vi "StopControl.vi"(6 "Loop Iteration":i32, 8 "Reset":bool, 9 "Rate (unit/s)":dbl=0.5, 11 "Motor Value":dbl step=0.1) -> (0 "Done Stopping":bool, 3 "New Motor Value":dbl)   [LabVIEW 2012]
doc: "Stops a given motor value based on time since last call and given rate. Rate of change is always linear with respect to time. Designed to be run multiple times in while loop. Use shift register to maintain Motor Value in external while loop."
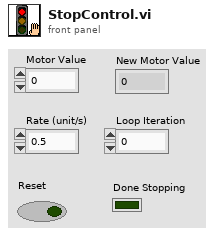
[diagram p1: front panel]
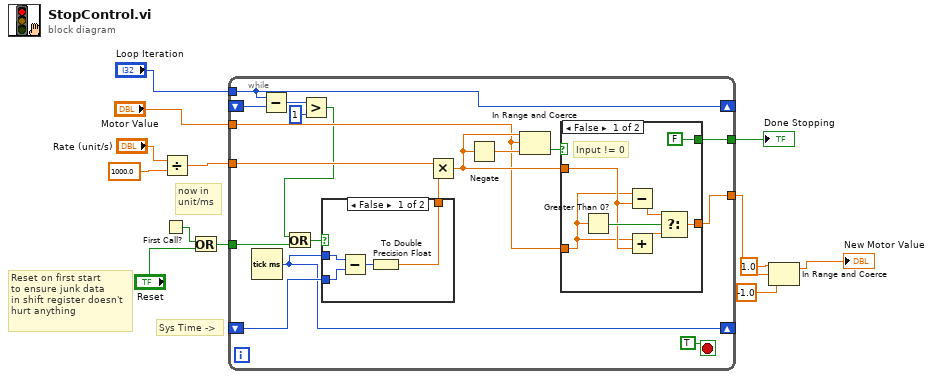
[diagram p0: block diagram]
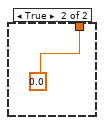
[diagram p2: hidden frame]
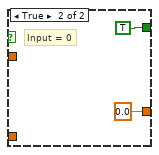
[diagram p3: hidden frame]
diagram:
  # "Sys Time ->"
  # "now in\nunit/ms"
  # "Reset on first start\nto ensure junk data\nin shift register doesn't\nhurt anything"
  n1 = First Call?() -> (First Call?: T/F=w9:bool)
  n2 = Divide(x="Rate (unit/s)", y=1000.0) -> (x/y=w10:dbl)
  n3 = Or(x=w9, y="Reset") -> (x .or. y?=w7:bool)
  n4 = while {
    tunnel: w10 -> [w29]
    tunnel: [w31] -> w13
    tunnel: w7 -> [w16]
    shift-right: [w22] -> _
    shift-left: _ -> [w23]
    tunnel: "Motor Value" -> [w26]
    tunnel: [w24] -> w5
    tunnel: "Loop Iteration" -> [w19]
    shift-right: [w19] -> _
    shift-left: _ -> [w18]
    stop <- TRUE stop-if-true
    n5 = Tick Count (ms)() -> (millisecond timer value=w22:u32)
    n6 = Subtract(x=w19, y=w18) -> (x-y=w20:i32)
    n7 = Greater?(x=w20, y=1) -> (0:w15:bool)
    n8 = Or(x=w15, y=w16) -> (x .or. y?=w14:bool)
    n9 = case shown="False" w14 {
      tunnel: w23 -> [w34 _]
      tunnel: w22 -> [w35 _]
      tunnel: [w32 0.0] -> w21
      frame False {
        n10 = Subtract(x=w35, y=w34) -> (x-y=w33:u32)
        n11 = To Double Precision Float(number=w33) -> (double precision float=w32:dbl)
      }
      frame True {
      }
    }
    n12 = Multiply(x=w29, y=w21) -> (x*y=w27:dbl)
    n13 = Negate(x=w27) -> (-x=w28:dbl)
    n14 = In Range and Coerce(upper limit=w27, x=w26, lower limit=w28) -> (In Range?=w25:bool)  [unwired: 1 out]
    n15 = case shown="False" w25 {
      tunnel: [w40 0.0] -> w24
      tunnel: w27 -> [w38 _]
      tunnel: w26 -> [w37 _]
      tunnel: [FALSE TRUE] -> w31
      frame False {
        # "Input != 0"
        n16 = Greater Than 0?(x=w37) -> (x > 0?=w42:bool)
        n17 = Subtract(x=w37, y=w38) -> (x-y=w41:dbl)
        n18 = Add(x=w37, y=w38) -> (x+y=w39:dbl)
        n19 = Select(t=w41, s=w42, f=w39) -> (s? t:f=w40:dbl)
      }
      frame True {
        # "Input = 0"
      }
    }
  }
  "Done Stopping" <- w13
  n20 = In Range and Coerce(upper limit=1.0, x=w5, lower limit=-1.0) -> (coerced(x)=→"New Motor Value":dbl)  [unwired: 1 out]
